vi "ReadKeithley6482.vi"(8 "Error In":errorcluster, 11 "Keithley 6482 In":refnum<visa-resource-name>[](array[refnum])) -> (0 "Error Out":errorcluster, 2 "Data":dbl[](array[numeric]), 3 "Keithley 6482 Out":refnum<visa-resource-name>[](array[refnum]))   [LabVIEW 2012]
uses:
  libs/Keithley-6482/Keithley-6482.lvlib
  libs/LV-Utilities/LV-Utilities.lvlib
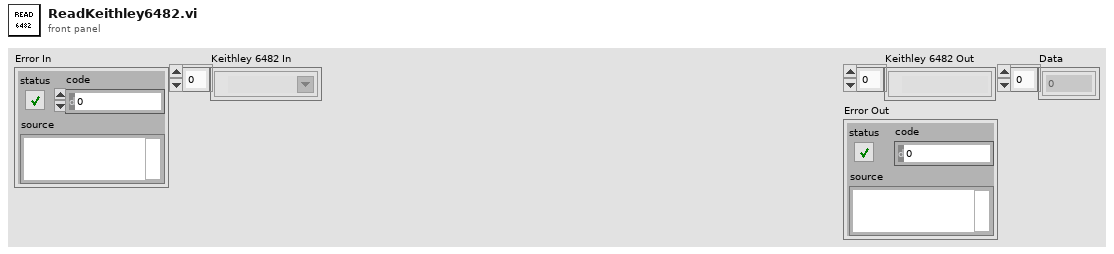
[diagram p1: front panel]
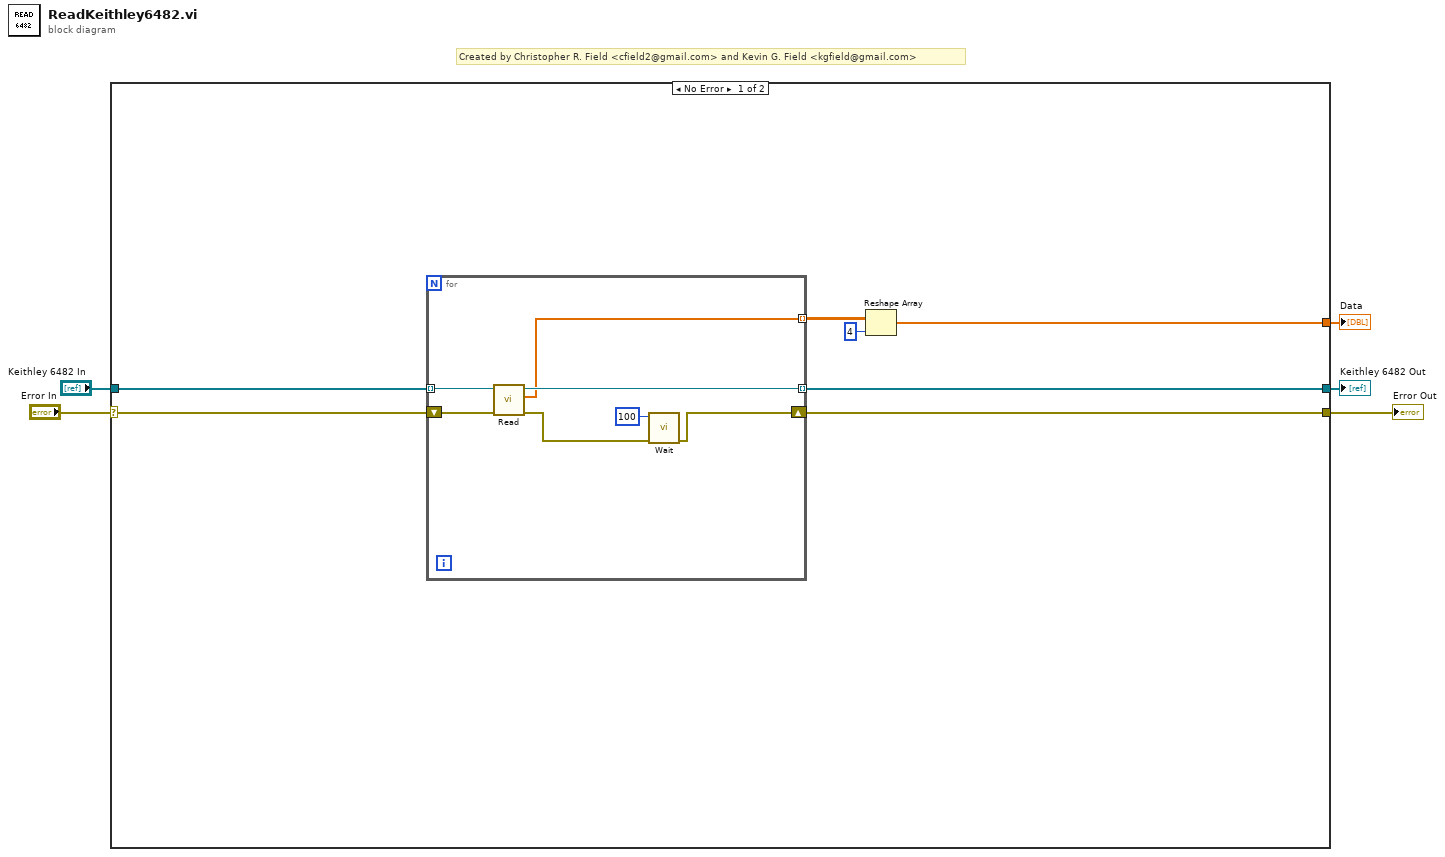
[diagram p0: block diagram]
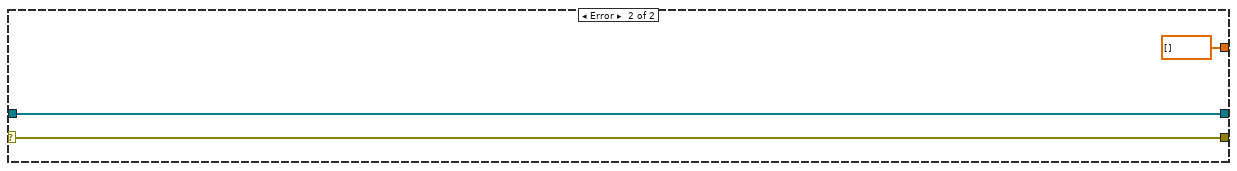
[diagram p2: hidden frame]
diagram:
  # "Created by Christopher R. Field <cfield2@gmail.com> and Kevin G. Field <kgfield@gmail.com>"
  n1 = case shown="No Error" "Error In" {
    selector: "Error In" -> [w10 w21]
    tunnel: "Keithley 6482 In" -> [w9 w22]
    tunnel: [w8 w22] -> w3
    tunnel: [w7 w21] -> w2
    tunnel: [w6 dbl[] [] ("Values")] -> w1
    frame No Error {
      n2 = for {
        tunnel: w9 -> [w19] mode=indexing
        tunnel: [w18] -> w8 mode=indexing
        shift-right: [w14] -> w7
        shift-left: w10 -> [w17]
        tunnel: [w16] -> w11 mode=indexing
        n3 = call "Read.vi"("Error In"=w17, "Keithley 6482 In"=w19) -> ("Error Out"=w15:errorcluster, "Values"=w16:dbl[], "Keithley 6482 Out"=w18:refnum<visa-resource-name>)  [unwired: 7 in]
        n4 = call "Wait.vi"("Error In"=w15, "Wait Time (msec)"=u32 100) -> ("Error Out"=w14:errorcluster)  [unwired: 9 in]
      }
      n5 = Reshape Array(w11, 4 ("dimension size")) -> (w6:dbl[])
    }
    frame Error {
    }
  }
  "Keithley 6482 Out" <- w3
  "Error Out" <- w2
  "Data" <- w1
